vi "Get Text Style Format.vi"(9 "Style Name":T1, 11 "[Named Text Styles]":T2[](array[typedef]) {"Text Formatting"."Font Size" min=6.0 step=1.0}) -> (1 "Found?":bool, 3 "Text Style":T2 {"Text Formatting"."Font Size" min=6.0 step=1.0})   [LabVIEW 2021, in "Notebook.lvlib"]
uses:
  Notebook.lvlib
  Rich Text Box/Named Text Style.ctl
  Rich Text Box/Text Formatting.ctl
  Rich Text Box/Text Colors.ctl
  Rich Text Box/Text Style.ctl
  Rich Text Box/Text Alignment.ctl
  Rich Text Box/Text Format List.ctl
  Rich Text Box/Rich Text Box.lvlib
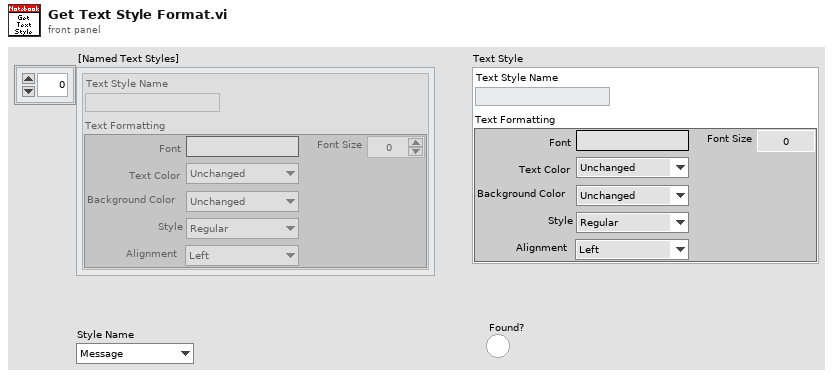
[diagram p1: front panel]
types:
  T1 = typedef "Notebook.lvlib/Text Format List.ctl" = enum16{"Message", "Result", "Error", "Setting", "Verbose", "Warning"}
  T2 = typedef "Notebook.lvlib/Named Text Style.ctl" = cluster{"Text Formatting":T3, "Text Style Name":string}
  T3 = typedef "Rich Text Box.lvlib/Text Formatting.ctl" = cluster{"Font":string, "Text Color":T4, "Background Color":T4, "Style":T5, "Font Size":dbl, "Alignment":T6}
  T4 = typedef "Rich Text Box.lvlib/Text Colors.ctl" = enum16{"Unchanged", "Black", "Blue", "Cyan", "Maroon", "Gray", "Violet", "Green", "Light Green", "Orange", "Yellow", "Magenta", "Red", "White"}
  T5 = typedef "Rich Text Box.lvlib/Text Style.ctl" = enum16{"Regular", "Bold", "Italic", "Underline", "Strikeout"}
  T6 = typedef "Rich Text Box.lvlib/Text Alignment.ctl" = enum16{"Left", "Right", "Center"}
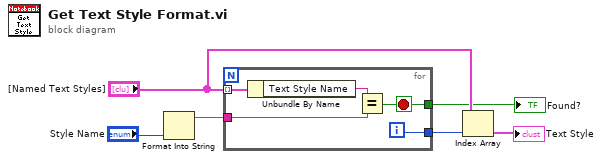
[diagram p0: block diagram]
diagram:
  n1 = Format Into String("Style Name") -> (resulting string=w5:string)  [unwired: 3 in, 1 out]
  n2 = for {
    tunnel: "[Named Text Styles]" -> [w11] mode=indexing
    tunnel: w5 -> [w9]
    tunnel: [w8] -> w4
    tunnel: [w7] -> w1
    i -> [w8]
    stop <- w7 stop-if-true
    n3 = Unbundle By Name(w11) -> ("Text Style Name"=w10:string)
    n4 = Equal?(x=w10, y=w9) -> (x = y?=w7:bool)
  }
  "Found?" <- w1
  n5 = Index Array(array="[Named Text Styles]", index=w4) -> (element=→"Text Style":T2)
